vi "Read Allele-Bit.vi"(8 "error in (no error)":errorcluster, 11 "Binary Gene in":refnum<class "Binary Gene.lvclass">) -> (0 "error out":errorcluster, 2 "Allele-Bit":T1, 3 "Binary Gene out":refnum<class "Binary Gene.lvclass">)   [LabVIEW 2016, in "Binary Gene.lvclass"]
uses:
  Binary Gene.lvclass
  _typedefs/BinaryGene_Allele.ctl
  Binary Gene.lvclass/Binary Gene.ctl
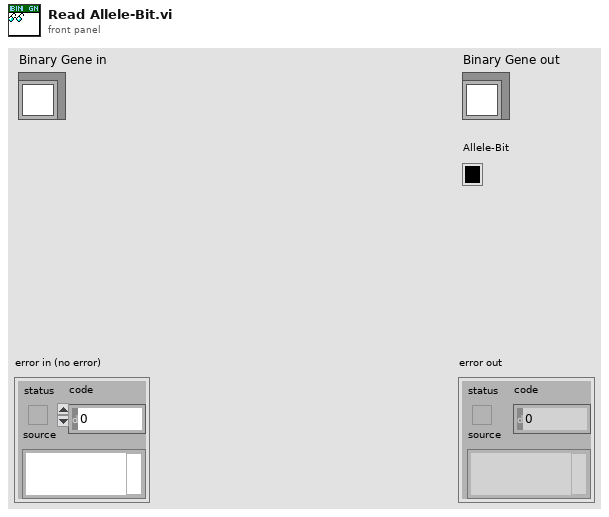
[diagram p1: front panel]
types:
  T1 = typedef "Binary Gene.lvclass/BinaryGene_Allele.ctl" = bool
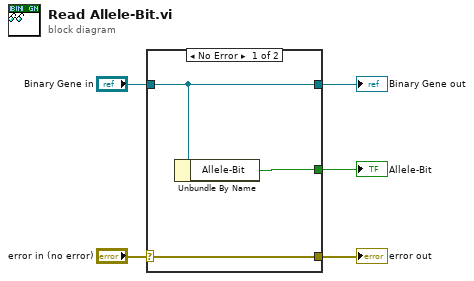
[diagram p0: block diagram]
diagram:
  n1 = case shown="No Error" "error in (no error)" {
    selector: "error in (no error)" -> [w8 w9]
    tunnel: [w8 w9] -> w4
    tunnel: [w7 w10] -> w2
    tunnel: "Binary Gene in" -> [w7 w10]
    tunnel: [w6 _] -> w1
    frame No Error {
      n2 = Unbundle By Name(w7) -> ("Allele-Bit"=w6:T1)
    }
    frame Error {
    }
  }
  "error out" <- w4
  "Binary Gene out" <- w2
  "Allele-Bit" <- w1
